vi "Create Table.vi"() -> ()   [LabVIEW 2015]
uses:
  <vilib>/addons/database/Connection.llb/DB Tools Open Connec (String).vi
  <vilib>/addons/database/Connection.llb/Conn Execute.vi
  <vilib>/addons/database/NI_Database_API.lvlib
  <vilib>/Utility/config.llb/NI_LVConfig.lvlib
panel:
  out "error out":errorcluster
  out "spreadsheet string":string
  in  "Listbox":i32(listbox)
  out "concatenated string 2":string
  out "concatenated string":string
  in  "Table Name":string
  in  "Table Name":string
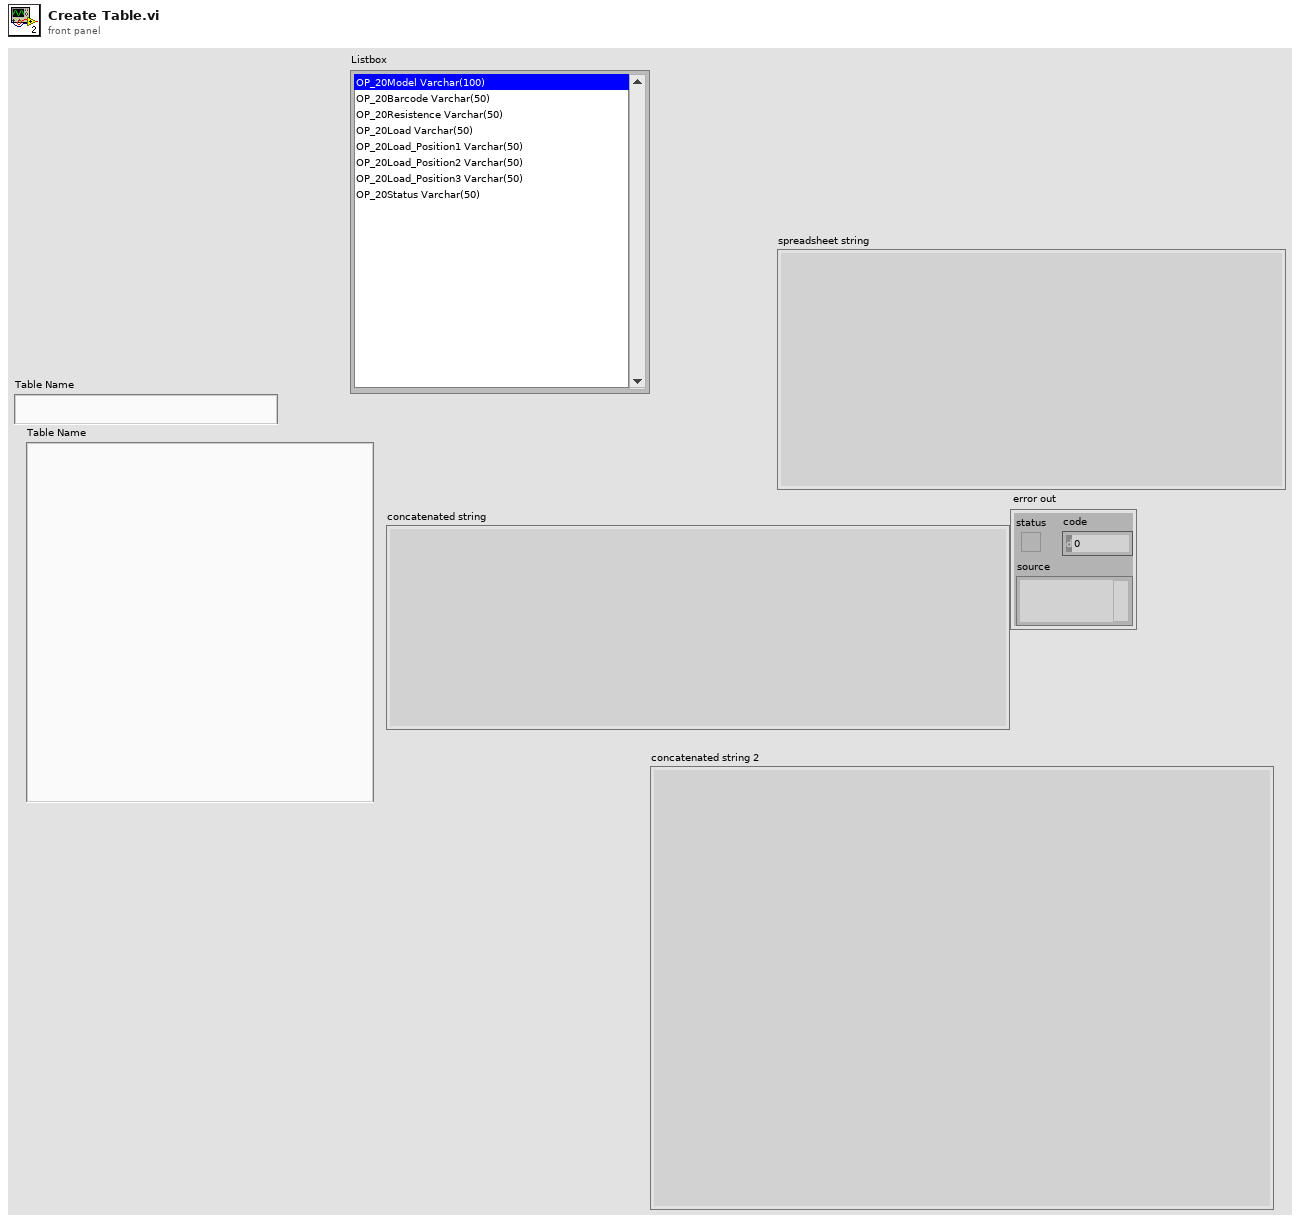
[diagram p1: front panel]
types:
  T1 = typedef "NI_LVConfig.lvlib/Config Data RefNum.ctl" = refnum<k1>
  T2 = typedef "NI_Database_API.lvlib/Conn ObjectReference.ctl" = refnum<k1>
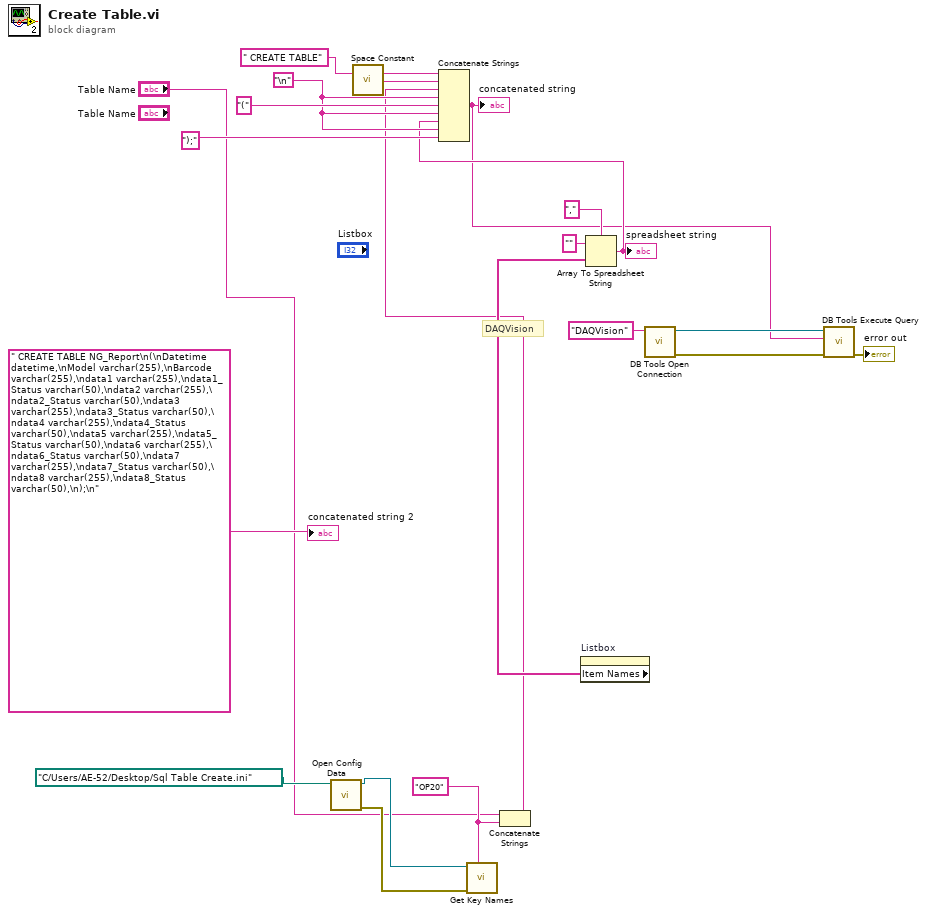
[diagram p0: block diagram]
diagram:
  w3 = "OP20" ("key")
  w19 = "\n"
  # "DAQVision"
  n1 = call <vilib>:"Open Config Data.vi"("configuration file path"=path "C:/Users/AE-52/Desktop/Sql Table Create.ini" ("base path")) -> ("error out"=w6:errorcluster, "refnum"=w7:T1)  [unwired: 8 in, 1 out]
  n2 = call <vilib>:"Space Constant.vi"() -> ("String"=w16:string)
  n3 = call <vilib>:"Get Key Names.vi"("section"=w3, "error in (no error)"=w6, "refnum"=w7) -> ()  [unwired: 5 in, 4 out]
  n4 = Concatenate Strings("Table Name", w3) -> (w1:string)
  n5 = property on="Listbox" class="LstBox (strict)"() -> ("Item Names"=w4:string[])  [unwired: 2 in, 2 out]
  n6 = Array To Spreadsheet String(delimiter (Tab)=",", array=w4, 3:"" ("format string")) -> (spreadsheet string=w10:string)
  "spreadsheet string" <- w10
  n7 = Concatenate Strings(" CREATE TABLE" ("string"), w16, w1, w19, "(" ("string"), w19, w10, w19, ");" ("string")) -> (w9:string)
  "concatenated string" <- w9
  n8 = call-poly <vilib>:"DB Tools Open Connection.vi"("connection information"="DAQVision" ("password")) -> ("error out"=w12:errorcluster, "connection reference"=w13:T2)  [unwired: 7 in]
  n9 = call-poly <vilib>:"DB Tools Execute Query.vi"("error in (no error)"=w12, "SQL query"=w9, "connection reference"=w13) -> ("error out"=→"error out":errorcluster)  [unwired: 5 in, 1 out]
  "concatenated string 2" <- " CREATE TABLE NG_Report\n(\nDatetime datetime,\nModel varchar(255),\nBarcode varchar(255),\ndata1 varchar(255),\ndata1_Status varchar(50),\ndata2 varchar(255),\ndata2_Status varchar(50),\ndata3 varchar(255),\ndata3_Status varchar(50),\ndata4 varchar(255),\ndata4_Status varchar(50),\ndata5 varchar(255),\ndata5_Status varchar(50),\ndata6 varchar(255),\ndata6_Status varchar(50),\ndata7 varchar(255),\ndata7_Status varchar(50),\ndata8 varchar(255),\ndata8_Status varchar(50),\n);\n" ("SQL query")
